vi "String Norm to Byte.vi"(1 "String In":string) -> (0 "Byte String Out":string)   [LabVIEW 2019]
panel:
  in  "delimeter":string="A"
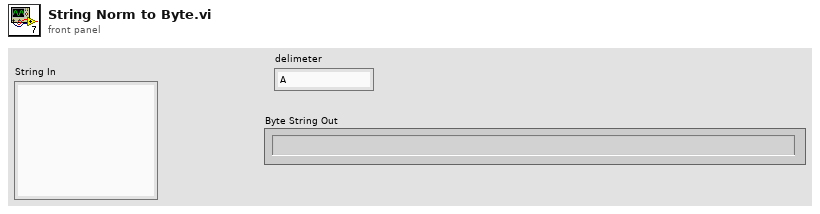
[diagram p1: front panel]
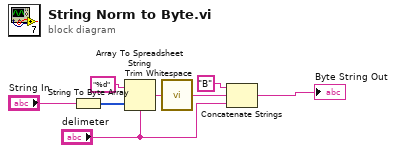
[diagram p0: block diagram]
diagram:
  n1 = String To Byte Array(string="String In") -> (unsigned byte array=w6:u8[])
  n2 = Array To Spreadsheet String(delimiter (Tab)="delimeter", array=w6, 3:"%d" ("format string")) -> (spreadsheet string=w3:string)
  n3 = call <vilib>:"Trim Whitespace.vi"("string"=w3) -> ("trimmed string"=w2:string)  [unwired: 1 in]
  n4 = Concatenate Strings("B" ("string"), w2, "delimeter") -> (→"Byte String Out":string)
